vi "Spy Flush Last Error.vi"(8 "error in (no error)":errorcluster, 11 "Mock Error Handler In":refnum<class "Mock Error Handler.lvclass">) -> (0 "error out":errorcluster, 1 "Errors":errorcluster, 2 "Message":string, 3 "Mock Error Handler Out":refnum<class "Mock Error Handler.lvclass">)   [LabVIEW 2020, in "Mock Error Handler.lvclass"]
doc: "Spys on errors sent to the error handler. This Method requires a lock on the execution thread to prevent race conditions when testing other processes using the error handler."
uses:
  Mock Error Handler.lvclass
  Mock Error Handler.lvclass/Mock Error Handler.ctl
  Private/Error Message Data.ctl
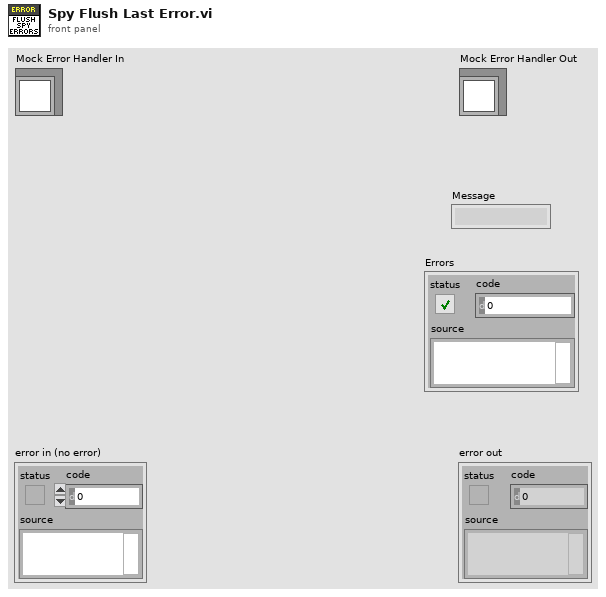
[diagram p1: front panel]
types:
  T1 = typedef "Mock Error Handler.lvclass/Error Message Data.ctl" = cluster{"Error Type":string, "Location":string, "Error":errorcluster}
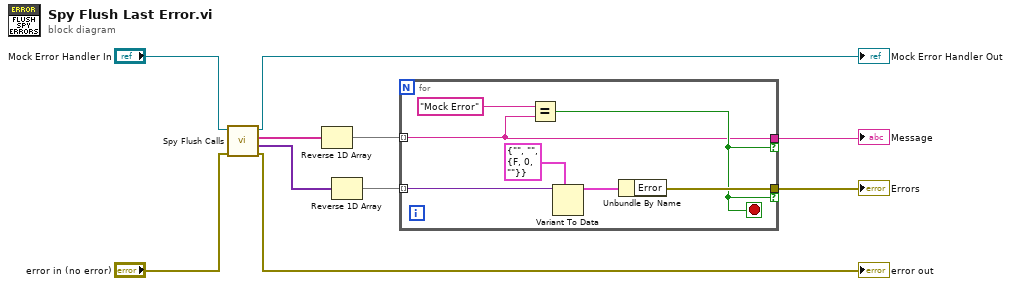
[diagram p0: block diagram]
diagram:
  n1 = call "Spy Flush Calls.vi"("error in (no error)"="error in (no error)", "Mock Process In"="Mock Error Handler In") -> ("error out"=→"error out":errorcluster, "Message Data"=w6:variant[], "Message"=w7:string[], "Mock Process Out"=→"Mock Error Handler Out":refnum<class "Mock Error Handler.lvclass">)  [unwired: 6 in]
  n2 = Reverse 1D Array(array=w7) -> (reversed array=w8:string[])
  n3 = Reverse 1D Array(array=w6) -> (reversed array=w5:variant[])
  n4 = for {
    tunnel: [w14] -> w10 if=w13
    tunnel: w8 -> [w12] mode=indexing
    tunnel: [w12] -> w9 if=w13
    tunnel: w5 -> [w11] mode=indexing
    stop <- w13 stop-if-true
    n5 = Equal?(x="Mock Error", y=w12) -> (x = y?=w13:bool)
    n6 = Variant To Data(type=T1 {"Error Type"="", "Location"="", "Error"={"status"=FALSE, "code"=0, "source"=""}} ("Error Message Data"), Variant=w11) -> (data=w16:T1)  [unwired: 1 in, 1 out]
    n7 = Unbundle By Name(w16) -> ("Error"=w14:errorcluster)
  }
  "Message" <- w9
  "Errors" <- w10
